vi "1D ANOVA.vi"(1 "# of levels":i32 format="%0.0f", 5 "Index":i32[](array[numeric]) format="%0.0f", 6 "X":dbl[](array[numeric]) format="%0.2f") -> (0 "sig A":dbl format="%0.4f", 2 "error":i32, 3 "tss":dbl format="%0.4f", 4 "msa":dbl format="%0.4f", 7 "f":dbl format="%0.4f", 8 "mse":dbl format="%0.4f", 9 "ssa":dbl format="%0.4f", 10 "sse":dbl format="%0.4f")   [LabVIEW 2017, in "NI_AALPro.lvlib"]
doc: "Takes an array, <B>X</B>, of experimental observations made at various <B>levels</B> of a factor, with at least one observation per level, and performs a one-way analysis of variance in the fixed effect model."
uses:
  NI_AALPro.lvlib
  <resource>/lvanlys.dll
panel:
  # "1D ANOVA"
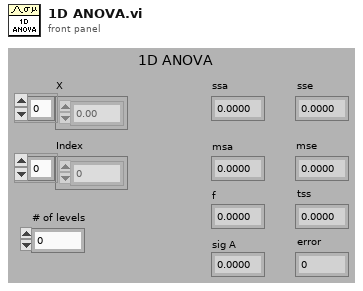
[diagram p1: front panel]
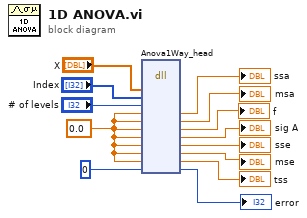
[diagram p0: block diagram]
diagram:
  w8 = 0.0
  n1 = dll-call lib="C:/Program Files (x86)/National Instruments/LabVIEW 2017/resource/lvanlys.*" fn="Anova1Way_head"("X"="X", "Index"="Index", "# of levels"="# of levels", "output param"=w8, "output param"=w8, "output param"=w8, "output param"=w8, "output param"=w8, "output param"=w8, "output param"=w8, "output param"=0) -> ("output param"=→"ssa":dbl, "output param"=→"msa":dbl, "output param"=→"f":dbl, "output param"=→"sig A":dbl, "output param"=→"sse":dbl, "output param"=→"mse":dbl, "output param"=→"tss":dbl, "output param"=→"error":i32)  [unwired: 7 in, 2 out]
